vi "NI VeriStand - Move Custom Device Item.vi"(7 "Highlight? (F)":bool, 8 "error in (no error)":errorcluster, 10 "New Parent Ref in":T1 format="%.0x", 11 "Item Ref in":T1 format="%.0x") -> (0 "error out":errorcluster, 3 "Item Ref out":T1 format="%.0x", 4 "Moved?":bool)   [LabVIEW 2020, in "Custom Device API.lvlib"]
doc: "Moves a custom device item to a new location within the custom device hierarchy. For example, you can use this VI to move a channel from one section to another. If you try to move an item to a location outside of its owning custom device, this VI returns an error."
uses:
  <vilib>/NI VeriStand/Custom Device API/Custom Device API.lvlib
  <vilib>/NI VeriStand/Custom Device API/Custom Device Item Ref.ctl
  c8d440cf-8dd2-4826-98f1-f9614a67f8cf.vi
  <vilib>/NI VeriStand/Custom Device API/Custom Device Offline Path.vi
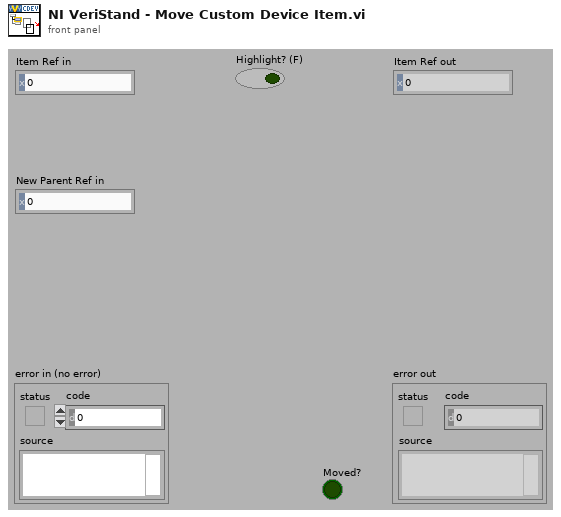
[diagram p1: front panel]
types:
  T1 = typedef "Custom Device API.lvlib/Custom Device Item Ref.ctl" = u64
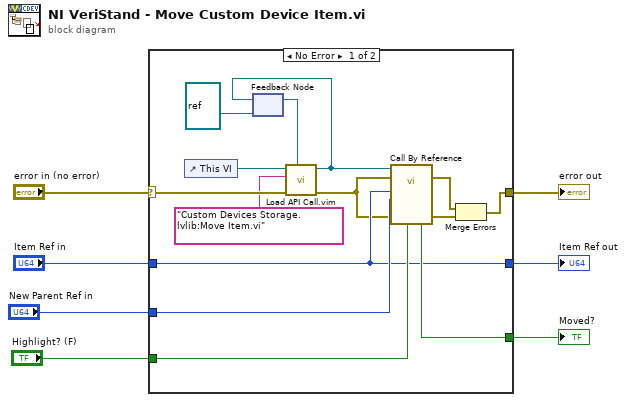
[diagram p0: block diagram]
diagram:
  n1 = case shown="No Error" "error in (no error)" {
    selector: "error in (no error)" -> [w13 w22]
    tunnel: [w20 w22] -> w7
    tunnel: "Item Ref in" -> [w16 w23]
    tunnel: [w16 w23] -> w5
    tunnel: [w19 _] -> w4
    tunnel: "Highlight? (F)" -> [w18 _]
    tunnel: "New Parent Ref in" -> [w17 _]
    frame No Error {
      n2 = control-ref of="This VI"() -> (w14:refnum<vi>)
      n3 = feedback #1(refnum<vi> refnum ("type specifier VI Refnum (for type only)")) -> (w15:refnum<vi>)
      n4 = call "Load API Call.vim"("VI reference in"=w15, "error in (no error)"=w13, "VI qualified name"="Custom Devices Storage.lvlib:Move Item.vi", "Caller VI ref"=w14) -> ("error out"=w12:errorcluster, "VI reference"=w11:refnum<vi>)  [unwired: 6 in]
      n5 = feedback-in #1(w11) -> ()
      n6 = call-by-ref "?"(reference=w11, error in=w12, "Highlight? (F)"=w18, 8:"error in (no error)"=w12, "New Parent Ref in"=w17, "Node Ref in"=w16) -> (error out=w8:errorcluster, 0:"error out"=w21:errorcluster, "Moved"=w19:bool)  [unwired: 5 in, 2 out]
      n7 = Merge Errors(w8, w21) -> (w20:errorcluster)
    }
    frame Error {
    }
  }
  "Item Ref out" <- w5
  "error out" <- w7
  "Moved?" <- w4
